vi "Get OSF Status.vi"(8 "error in (no error)":errorcluster, 10 "Stop checjking if OK":bool, 11 "Log Record in":refnum<class "Log Record.lvclass">) -> (0 "error out":errorcluster, 3 "Log Record out":refnum<class "Log Record.lvclass">)   [LabVIEW 2020, in "Log Record.lvclass"]
uses:
  Log Record.lvclass
  <vilib>/ActorFramework/Time-Delayed Send Message/Time-Delay Override Options.ctl
  Log Record.lvclass/Log Record.ctl
panel:
  out "current time":timestamp
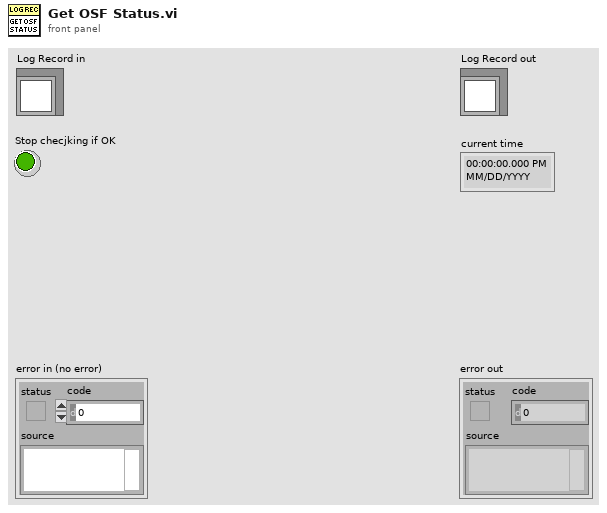
[diagram p1: front panel]
types:
  T1 = typedef "Time-Delay Override Options.ctl" = enum16{"Send next copy now", "Skip next scheduled copy", "Send next copy now and stop all further copies", "Stop all further copies"}
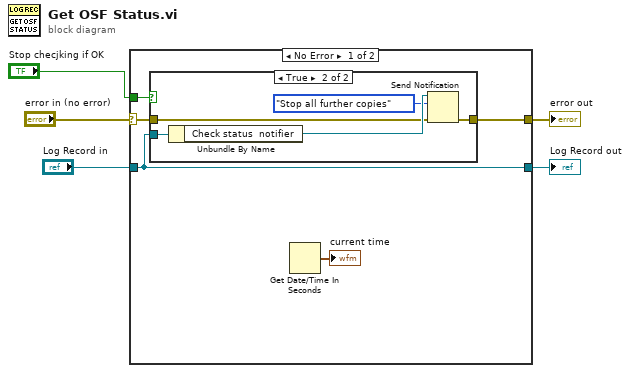
[diagram p0: block diagram]
diagram:
  n1 = case shown="No Error" "error in (no error)" {
    selector: "error in (no error)" -> [w9 w18]
    tunnel: [w8 w18] -> w4
    tunnel: [w10 w17] -> w2
    tunnel: "Log Record in" -> [w10 w17]
    tunnel: "Stop checjking if OK" -> [w7 _]
    frame No Error {
      n2 = case shown="True" w7 {
        tunnel: w10 -> [_ w16]
        tunnel: w9 -> [w11 w13]
        tunnel: [w11 w12] -> w8
        frame False {
        }
        frame True {
          n3 = Unbundle By Name(w16) -> ("Check status  notifier"=w15:refnum<notifier>)
          n4 = Send Notification(notification=Time-Delay_Override_Options."Stop all further copies", notifier=w15, error in (no error)=w13) -> (error out=w12:errorcluster)  [unwired: 1 out]
        }
      }
      n5 = Get Date/Time In Seconds() -> (seconds since 1Jan1904=→"current time":timestamp)
    }
    frame Error {
    }
  }
  "error out" <- w4
  "Log Record out" <- w2
